vi "DSF.Engine.Transceiver Thread.Get Thread ID Pool.vi"(11 "Transceiver Thread in":refnum<class "DSF.Engine.Transceiver Thread.lvclass">) -> (2 "Thread ID Pool":refnum<class "DSF.Engine.Pool.ID.lvclass">, 3 "Transceiver Thread out":refnum<class "DSF.Engine.Transceiver Thread.lvclass">)   [LabVIEW 2017, in "DSF.Engine.lvlib" / "DSF.Engine.Transceiver Thread.lvclass"]
uses:
  DSF.Engine.Transceiver Thread.lvclass
  Thread Pool/DSF.Engine.Pool.ID.lvclass
  DSF.Engine.Transceiver Thread.lvclass/DSF.Engine.Transceiver Thread.ctl
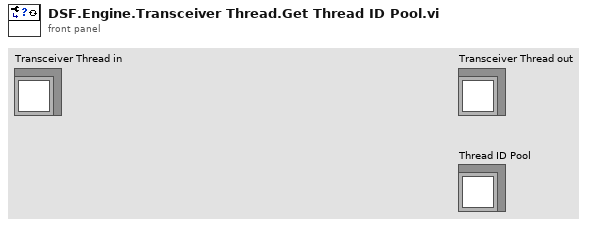
[diagram p1: front panel]
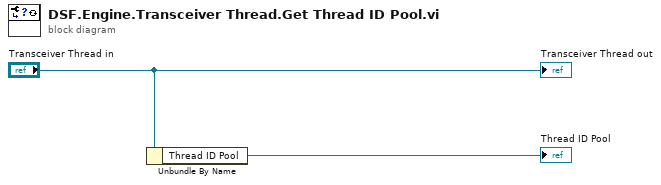
[diagram p0: block diagram]
diagram:
  n1 = Unbundle By Name("Transceiver Thread in") -> ("Thread ID Pool"=→"Thread ID Pool":refnum<class "DSF.Engine.Pool.ID.lvclass">)
  "Transceiver Thread out" <- "Transceiver Thread in"
